vi "draw.vi"(0 "reference":refnum<class "NoteNode.lvclass">, 1 "graphics":refnum<class "Graphics.lvclass">, 5 "error in (no error)":errorcluster) -> (14 "reference out":refnum<class "NoteNode.lvclass">, 19 "error out":errorcluster)   [LabVIEW 2012, in "NoteNode.lvclass"]
doc: "public void draw(Graphics2D g2)"
uses:
  <resource>/Framework/Providers/Open_GDS/UML/NoteNode_class/NoteNode.lvclass
  <resource>/Framework/Providers/Open_GDS/UML/Graphics_class/Graphics.lvclass
  <resource>/Framework/Providers/Open_GDS/UML/MultiLineString_class/MultiLineString.lvclass
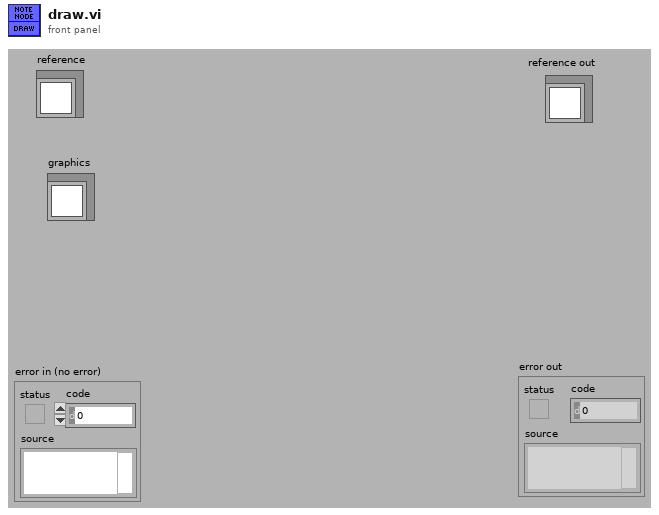
[diagram p1: front panel]
types:
  T1 = typedef "NoteNode.lvclass/ObjectAttributes.ctl" = cluster{"Base class":T2, "DEFAULT_WIDTH":i32, "DEFAULT_HEIGHT":i32, "DEFAULT_COLOR":u32, "FOLD_X":i32, "FOLD_Y":i32, "color":u32, "text":refnum<class "MultiLineString.lvclass">, "pointNodes":refnum<class "AbstractNode.lvclass">[]}
  T2 = typedef "RectangularNode.lvclass/ObjectAttributes.ctl" = cluster{"Base class":T3, "bounds":T4}
  T3 = typedef "AbstractNode.lvclass/ObjectAttributes.ctl" = cluster{"parent":refnum<class "AbstractNode.lvclass">, "children":refnum<class "AbstractNode.lvclass">[], "Hidden":bool}
  T4 = typedef "Rectangle Rectangle2D.ctl" = cluster{"x":dbl, "y":dbl, "width":dbl, "height":dbl}
  T5 = typedef "Point Point2D.ctl" = cluster{"x":dbl, "y":dbl}
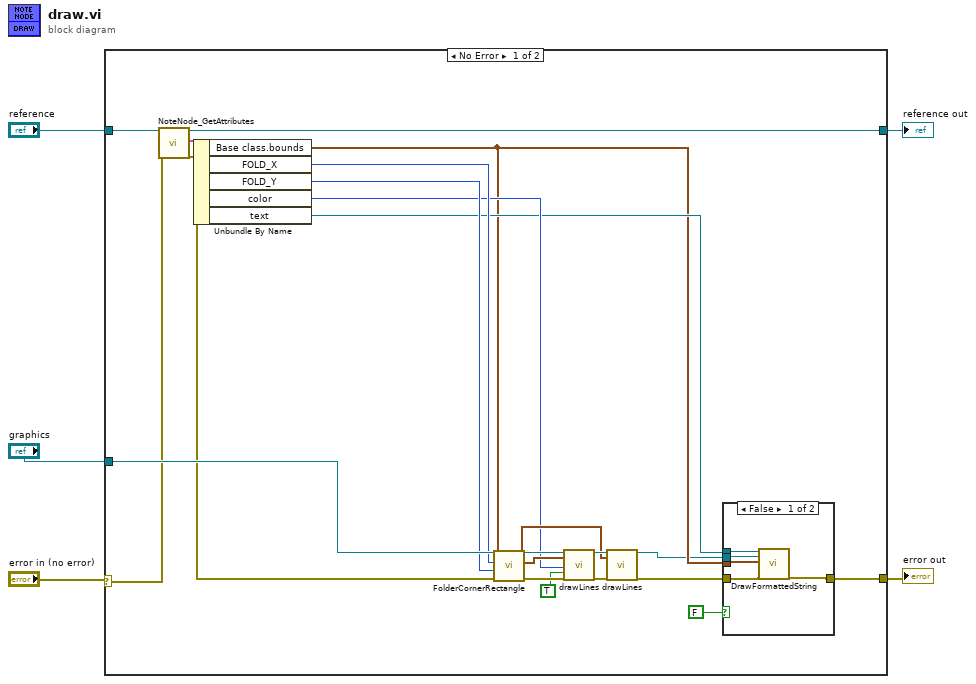
[diagram p0: block diagram]
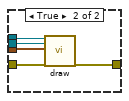
[diagram p2: hidden frame]
diagram:
  n1 = case shown="No Error" "error in (no error)" {
    selector: "error in (no error)" -> [w9 w37]
    tunnel: "reference" -> [w26 w38]
    tunnel: [w25 w37] -> w4
    tunnel: [w24 w38] -> w3
    tunnel: "graphics" -> [w23 _]
    frame No Error {
      n2 = call <resource>:"NoteNode_GetAttributes.vi"("reference in"=w26, "error in (no error)"=w9) -> ("reference out"=w24:refnum<class "NoteNode.lvclass">, "Attributes"=w22:T1, "error out"=w21:errorcluster)  [unwired: 15 out]
      n3 = Unbundle By Name(w22) -> ("Base class.bounds"=w8:T4, "FOLD_X"=w20:i32, "FOLD_Y"=w19:i32, "color"=w14:u32, "text"=w13:refnum<class "MultiLineString.lvclass">)
      n4 = call <resource>:"FolderCornerRectangle.vi"("error out 2"=w21, "FOLD_Y"=w19, "FOLD_X"=w20, "bounds"=w8) -> ("error out"=w11:errorcluster, "Array 2"=w18:T5[], "Array"=w15:T5[])  [unwired: 5 out]
      n5 = call <resource>:"drawLines.vi"("reference"=w23, "points"=w18, "color(if not used=default color)"=w14, "fill?(F)"=TRUE, "error in (no error)"=w11) -> ("reference out"=w17:refnum<class "Graphics.lvclass">, "error out"=w16:errorcluster)  [unwired: 2 in, 11 out]
      n6 = call <resource>:"drawLines.vi"("reference"=w17, "points"=w15, "error in (no error)"=w16) -> ("reference out"=w7:refnum<class "Graphics.lvclass">, "error out"=w12:errorcluster)  [unwired: 4 in, 11 out]
      n7 = case shown="False" FALSE {
        tunnel: [w29 w36] -> w25
        tunnel: w13 -> [w31 w35]
        tunnel: w12 -> [w30 w34]
        tunnel: w8 -> [w27 w33]
        tunnel: w7 -> [w28 w32]
        frame False {
          n8 = call-dynamic "DrawFormattedString.vi"("reference"=w31, "graphics"=w28, "bounds"=w27, "error in (no error)"=w30) -> ("error out"=w29:errorcluster)  [unwired: 14 in, 1 out]
        }
        frame True {
          n9 = call-dynamic "draw.vi"("reference"=w35, "graphics"=w32, "bounds"=w33, "error in (no error)"=w34) -> ("error out"=w36:errorcluster)  [unwired: 14 in, 1 out]
        }
      }
    }
    frame Error {
    }
  }
  "reference out" <- w3
  "error out" <- w4
